vi "Inst_DS360.vi"(8 "error in":errorcluster, 10 "All Message Queues in":T1, 11 "Prueba31 in":refnum<class "Prueba31.lvclass">) -> (0 "error out":errorcluster)   [LabVIEW 2019, in "Prueba31.lvclass"]
uses:
  Prueba31.lvclass
  QMH/Message Queue/All Message Queues.ctl
  QMH/Message Queue/Message Cluster.ctl
  Prueba31.lvclass/Prueba31.ctl
  <vilib>/Utility/error.llb/Error Cluster From Error Code.vi
  QMH/Message Queue/Enqueue Message (Single).vi
  <vilib>/ErrorRing/Error Ring.xnode
  QMH/Message Queue/Message Queue.lvlib
  Instrumento/DS360/DS360.lvclass
panel:
  out "All States":string[](array[string])
  out "Actual State":string
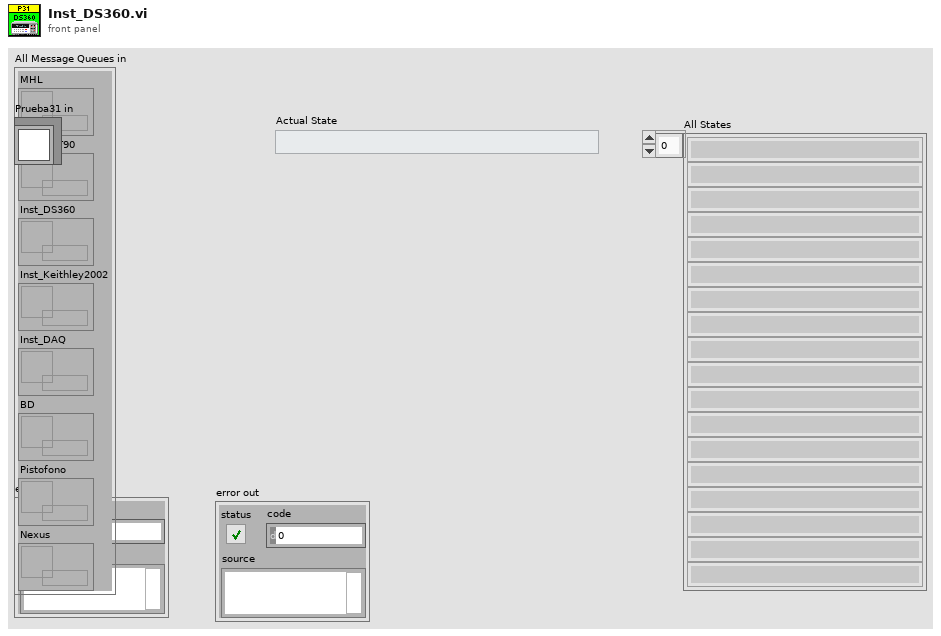
[diagram p1: front panel]
types:
  T1 = typedef "Message Queue.lvlib/All Message Queues.ctl" = cluster{"MHL":refnum<queue>, "Inst_CNT90":refnum<queue>, "Inst_DS360":refnum<queue>, "Inst_Keithley2002":refnum<queue>, "Inst_DAQ":refnum<queue>, "BD":refnum<queue>, "Pistofono":refnum<queue>, "Nexus":refnum<queue>}
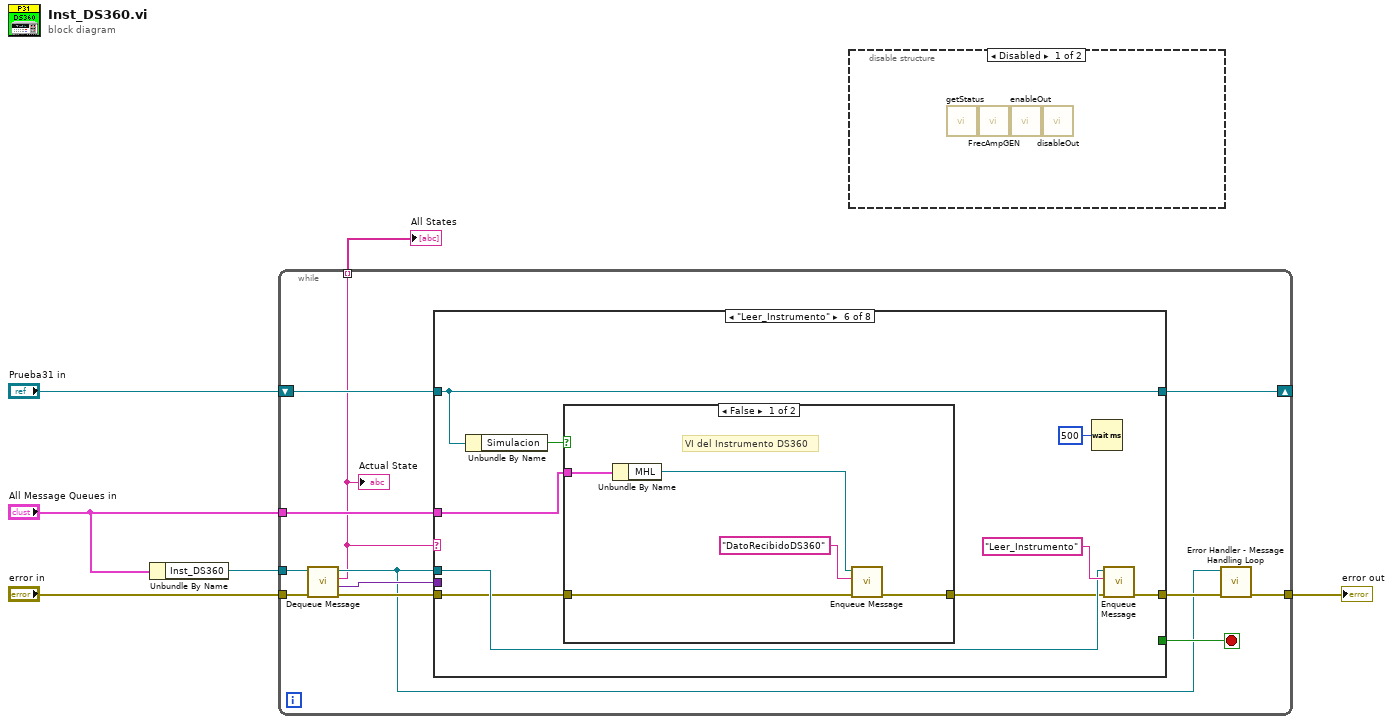
[diagram p0: block diagram]
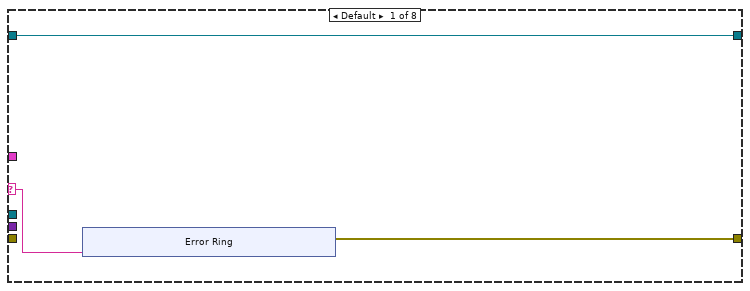
[diagram p3: hidden frame]
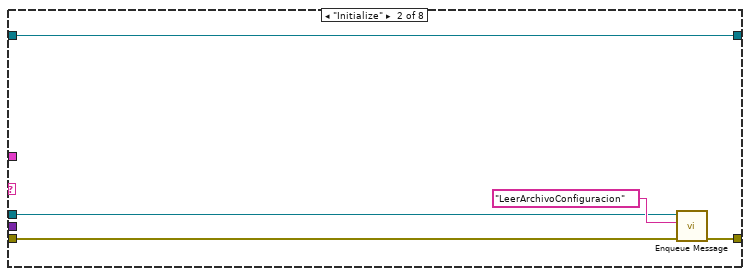
[diagram p4: hidden frame]
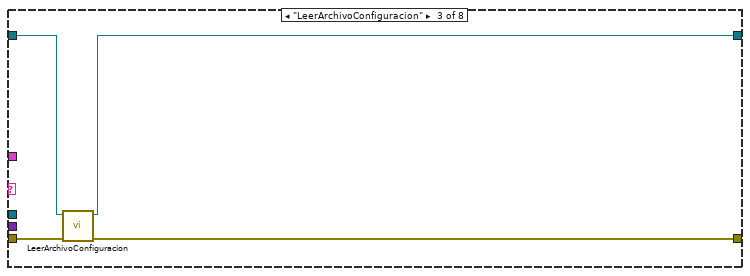
[diagram p5: hidden frame]
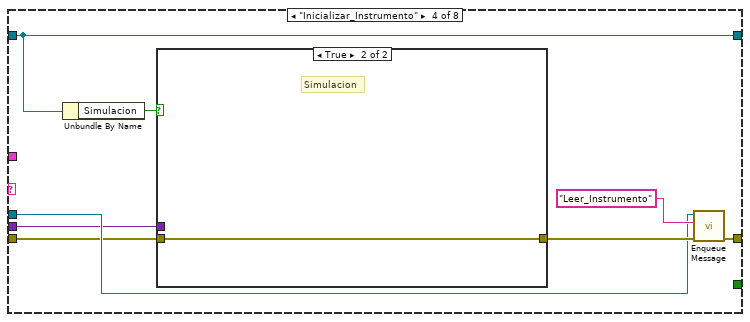
[diagram p6: hidden frame]
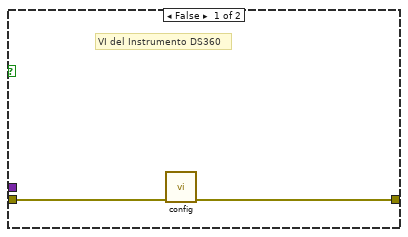
[diagram p7: hidden frame]
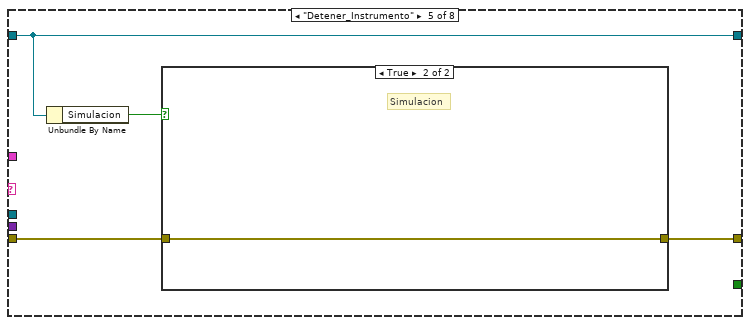
[diagram p8: hidden frame]
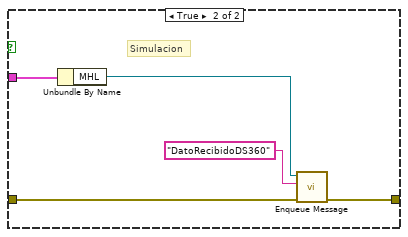
[diagram p10: hidden frame]
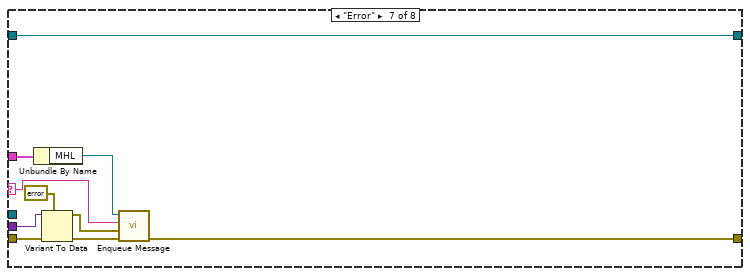
[diagram p11: hidden frame]
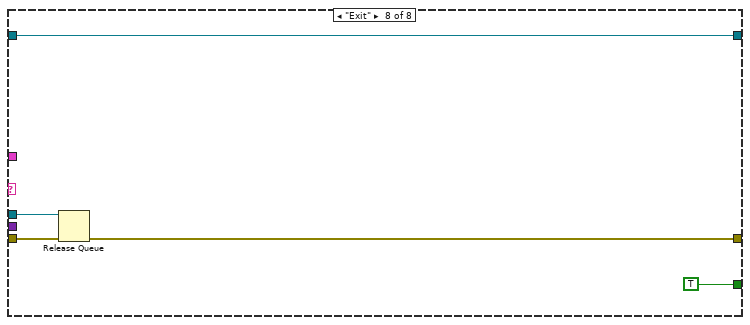
[diagram p12: hidden frame]
diagram:
  n1 = Unbundle By Name("All Message Queues in") -> ("Inst_DS360"=w4:refnum<queue>)
  n2 = while {
    tunnel: "error in" -> [w18]
    tunnel: w4 -> [w17]
    tunnel: "All Message Queues in" -> [w16]
    tunnel: [w9] -> w2
    shift-right: [w12] -> _
    shift-left: "Prueba31 in" -> [w15]
    tunnel: [w7] -> w1 mode=indexing
    stop <- w11 stop-if-true
    n3 = call "Dequeue Message.vi"("error in (no error)"=w18, "Message Queue"=w17) -> ("error out"=w13:errorcluster, "Message Data"=w14:variant, "Message"=w7:string, "dup Message Queue"=w8:refnum<queue>)  [unwired: 6 in]
    "Actual State" <- w7
    n4 = case shown="\"Leer_Instrumento\"" w7 {
      selector: w7 -> [w21 _ _ _ _ _ w76 _]
      tunnel: w16 -> [_ _ _ _ _ w57 w75 _]
      tunnel: w15 -> [w19 w33 w34 w42 w51 w56 w83 w85]
      tunnel: w8 -> [_ w29 _ w41 _ w60 _ w87]
      tunnel: w14 -> [_ _ _ w40 _ _ w80 _]
      tunnel: w13 -> [_ w30 w36 w39 w49 w58 w81 w88]
      tunnel: [w20 w31 w37 w38 w52 w61 w78 w84] -> w10
      tunnel: [w19 w33 w35 w42 w51 w56 w83 w85] -> w12
      tunnel: [_ _ _ _ _ _ _ TRUE] -> w11
      frame Default {
        n5 = xnode "Error Ring"("parameter 0"=w21) -> ("error out"=w20:errorcluster)
      }
      frame "Initialize" {
        n6 = call-poly "Enqueue Message.vi"("error in (no error)"=w30, "Message"="LeerArchivoConfiguracion", "Message Queue"=w29) -> ("error out"=w31:errorcluster)  [unwired: 7 in, 1 out]
      }
      frame "LeerArchivoConfiguracion" {
        n7 = call "LeerArchivoConfiguracion.vi"("error in"=w36, "Prueba31 in"=w34) -> ("error out"=w37:errorcluster, "Prueba31 out"=w35:refnum<class "Prueba31.lvclass">)  [unwired: 8 in]
      }
      frame "Inicializar_Instrumento" {
        n8 = Unbundle By Name(w42) -> ("Simulacion"=w44:bool)
        n9 = case shown="True" w44 {
          tunnel: [w47 w48] -> w45
          tunnel: w39 -> [w46 w48]
          tunnel: w40 -> [_ _]
          frame False {
            # "VI del Instrumento DS360"
            n10 = call "config.vi"("error in (no error)"=w46) -> ("error out"=w47:errorcluster)  [unwired: 9 in, 1 out]
          }
          frame True {
            # "Simulacion"
          }
        }
        n11 = call-poly "Enqueue Message.vi"("error in (no error)"=w45, "Message"="Leer_Instrumento", "Message Queue"=w41) -> ("error out"=w38:errorcluster)  [unwired: 7 in, 1 out]
      }
      frame "Detener_Instrumento" {
        n12 = Unbundle By Name(w51) -> ("Simulacion"=w50:bool)
        n13 = case shown="True" w50 {
          tunnel: [w53 w54] -> w52
          tunnel: w49 -> [w53 w54]
          frame False {
            # "Se cierra la comunicacion con los VI del\ninstrumento DS360"
          }
          frame True {
            # "Simulacion"
          }
        }
      }
      frame "Leer_Instrumento" {
        n14 = Unbundle By Name(w56) -> ("Simulacion"=w55:bool)
        n15 = case shown="False" w55 {
          tunnel: [w67 w72] -> w59
          tunnel: w58 -> [w64 w69]
          tunnel: w57 -> [w66 w71]
          frame False {
            # "VI del Instrumento DS360"
            n16 = Unbundle By Name(w66) -> ("MHL"=w65:refnum<queue>)
            n17 = call-poly "Enqueue Message.vi"("error in (no error)"=w64, "Message"="DatoRecibidoDS360", "Message Queue"=w65) -> ("error out"=w67:errorcluster)  [unwired: 7 in, 1 out]
          }
          frame True {
            # "Simulacion"
            n18 = Unbundle By Name(w71) -> ("MHL"=w70:refnum<queue>)
            n19 = call-poly "Enqueue Message.vi"("error in (no error)"=w69, "Message"="DatoRecibidoDS360", "Message Queue"=w70) -> ("error out"=w72:errorcluster)  [unwired: 7 in, 1 out]
          }
        }
        n20 = Wait (ms)(milliseconds to wait=u32 500) -> ()  [unwired: 1 out]
        n21 = call-poly "Enqueue Message.vi"("error in (no error)"=w59, "Message"="Leer_Instrumento", "Message Queue"=w60) -> ("error out"=w61:errorcluster)  [unwired: 7 in, 1 out]
      }
      frame "Error" {
        n22 = Unbundle By Name(w75) -> ("MHL"=w74:refnum<queue>)
        n23 = Variant To Data(error in=w81, type=errorcluster {"status"=FALSE, "code"=0, "source"=""} ("error constant"), Variant=w80) -> (data=w77:errorcluster, error out=w79:errorcluster)
        n24 = call-poly "Enqueue Message.vi"("error in (no error)"=w79, "Message Data"=w77, "Message"=w76, "Message Queue"=w74) -> ("error out"=w78:errorcluster)  [unwired: 6 in, 1 out]
      }
      frame "Exit" {
        n25 = Release Queue(queue=w87, error in (no error)=w88) -> (error out=w84:errorcluster)  [unwired: 1 in, 2 out]
      }
    }
    n26 = call "Error Handler - Message Handling Loop.vi"("error in (no error)"=w10, "Message Queue"=w8) -> ("dup error in"=w9:errorcluster)  [unwired: 8 in, 1 out]
  }
  "error out" <- w2
  "All States" <- w1
  n27 = disable-structure shown="Disabled" {
    frame Disabled {
      n28 = call "getStatus.vi"() -> ()  [unwired: 9 in, 3 out]
      n29 = call "FrecAmpGEN.vi"() -> ()  [unwired: 10 in, 2 out]
      n30 = call "enableOut.vi"() -> ()  [unwired: 10 in, 2 out]
      n31 = call "disableOut.vi"() -> ()  [unwired: 10 in, 2 out]
    }
    frame Enabled {
    }
  }
